vi "Non Linear Decimation XY.vi"(6 "Width":u32, 8 "error in (no error)":errorcluster, 9 "Xmin":dbl format="%#_13g", 10 "Xmax":dbl format="%#_13g", 11 "Data to Decimate":cluster{"X":dbl[], "Y":dbl[]}[](array[cluster])) -> (0 "error out":errorcluster, 3 "Decimated Data":cluster{"X":dbl[], "Y":dbl[]}[](array[cluster]))   [LabVIEW 2022 SP3, in "Decimation.lvlib"]
doc: "Decimate XY array to optimize the density of points per pixel to 2 : Min & Max per pixel."
uses:
  Decimation.lvlib
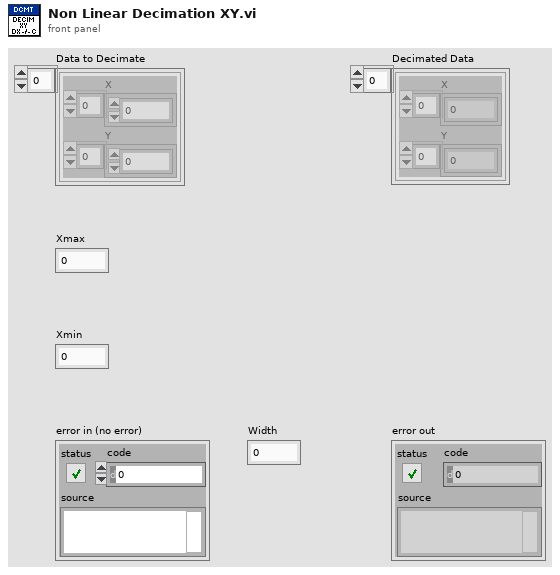
[diagram p1: front panel]
types:
  T1 = cluster{"Decimated Data":dbl[], "Decimated Data":dbl[]}
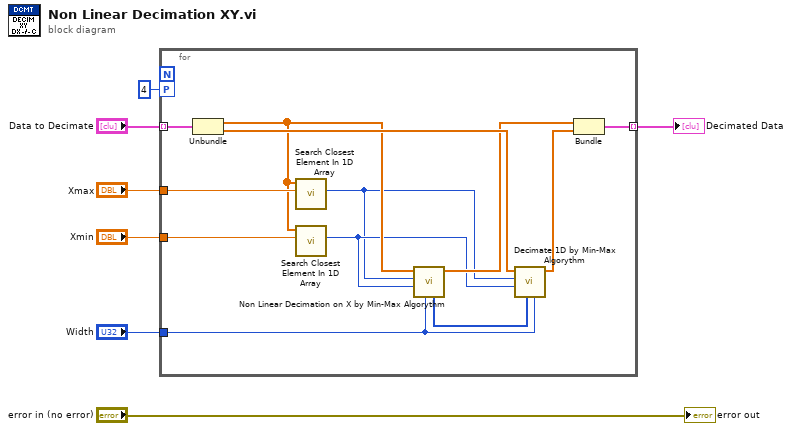
[diagram p0: block diagram]
diagram:
  n1 = for {
    tunnel: "Data to Decimate" -> [w19] mode=indexing
    tunnel: [w18] -> w5 mode=indexing
    tunnel: "Width" -> [w8]
    tunnel: "Xmax" -> [w14]
    tunnel: "Xmin" -> [w13]
    workers-P: 4 -> [_]
    n2 = Unbundle(w19) -> ("X"=w12:dbl[], "Y"=w17:dbl[])
    n3 = call "Search Closest Element In 1D Array.vi"("Desired element"=w14, "1D Array"=w12) -> ("Closest Index"=w9:i32)  [unwired: 8 in, 1 out]
    n4 = call "Search Closest Element In 1D Array.vi"("Desired element"=w13, "1D Array"=w12) -> ("Closest Index"=w10:i32)  [unwired: 8 in, 1 out]
    n5 = call "Non Linear Decimation on X by Min-Max Algorythm.vi"("Width"=w8, "Min Index"=w10, "Max Index"=w9, "Data To Decimate"=w12) -> ("Decimated Data"=w15:dbl[], "Packet size"=w11:i32[])  [unwired: 5 in, 1 out]
    n6 = call "Decimate 1D by Min-Max Algorythm.vi"("Width"=w8, "Packet sizes"=w11, "Min Index"=w10, "Max Index"=w9, "Data To Decimate"=w17) -> ("Decimated Data"=w16:dbl[])  [unwired: 5 in, 1 out]
    n7 = Bundle("Decimated Data"=w15, "Decimated Data"=w16) -> (w18:T1)  [unwired: 1 in]
  }
  "Decimated Data" <- w5
  "error out" <- "error in (no error)"
